vi "FileProducer.vi"(3 "Source File":path=path "C:/ScopeBinaryData.bin", 4 "error in (no error)":errorcluster, 5 "# Channels":i32, 6 "Samples per Channel":i32, 7 "Data Queue":refnum<queue>) -> (0 "error out":errorcluster)   [LabVIEW 2013]
uses:
  Execution Control Global.vi
panel:
  in  "Array":dbl[][](array[numeric])
  out "Data":dbl[][](graph)
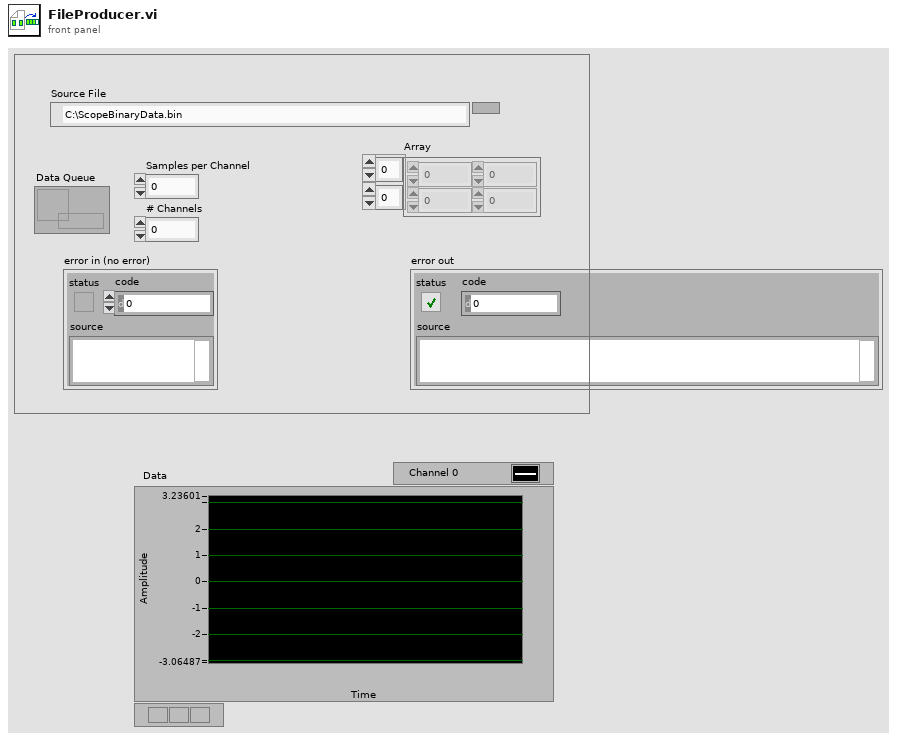
[diagram p1: front panel]
types:
  T1 = enum16{"open", "replace", "create", "open or create", "replace or create", "replace or create with confirmation"}
  T2 = enum16{"big-endian, network order", "native, host order", "little-endian"}
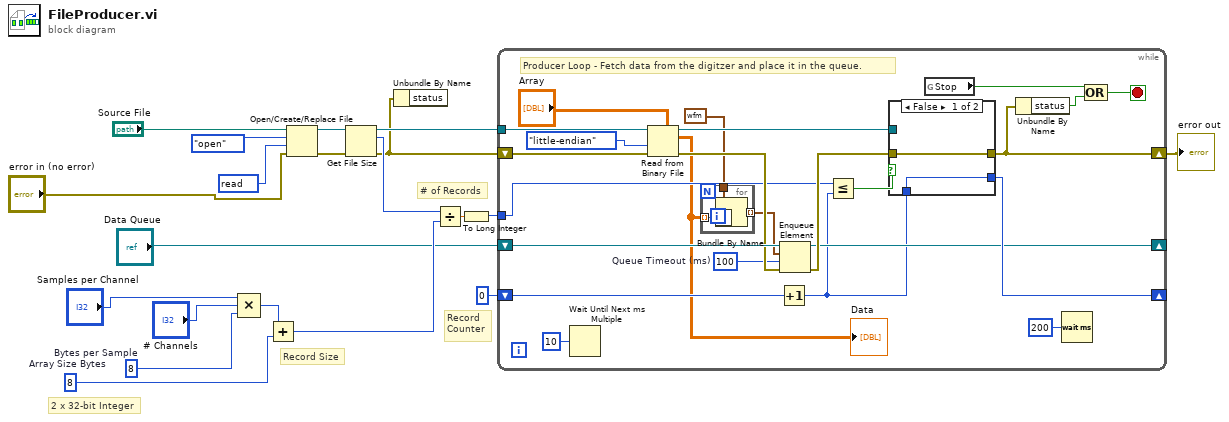
[diagram p0: block diagram]
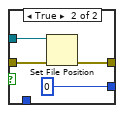
[diagram p2: hidden frame]
diagram:
  w13 = 8  # Array Size Bytes
  w12 = 8  # Bytes per Sample
  w4 = u32 2147483648 items=["read"=2147483648, "write"=1073741824, "read & write"=3221225472, "execute"=536870912, "all"=268435456] ("desired access (read & write)")
  # "# of Records"
  # "Record\nCounter"
  # "Record Size"
  # "2 x 32-bit Integer"
  n1 = Compound Arithmetic op=MULTIPLY("Samples per Channel", "# Channels", w12) -> (w11:i32)
  n2 = Add(x=w11, y=w13) -> (x+y=w10:i32)
  n3 = Open/Create/Replace File(file path (use dialog)="Source File", error in="error in (no error)", operation (0:open)=T1."open", access (0:read/write)=w4) -> (refnum out=w7:refnum<file>, error out=w8:errorcluster)  [unwired: 2 in, 1 out]
  n4 = Get File Size(file=w7, error in=w8) -> (refnum out=w20:refnum<file>, size (in bytes)=w19:i64, 0:w2:errorcluster)
  n5 = Unbundle By Name(w2) -> ()  [unwired: 1 out]
  n6 = Divide(x=w19, y=w10) -> (x/y=w18:dbl)
  n7 = To Long Integer(number=w18) -> (32bit integer=w17:i32)
  n8 = while {
    shift-right: [w40] -> w16
    shift-left: w2 -> [w41]
    tunnel: w20 -> [w42]
    shift-right: [w38] -> _
    shift-left: 0 -> [w26]
    tunnel: w17 -> [w28]
    shift-right: [w34] -> _
    shift-left: "Data Queue" -> [w37]
    stop <- w33 stop-if-true
    w31 = 100  # Queue Timeout (ms)
    # "Producer Loop - Fetch data from the digitzer and place it in the queue."
    n9 = Wait Until Next ms Multiple(millisecond multiple=u32 10) -> ()  [unwired: 1 out]
    n10 = Read from Binary File(5:"Array", 8:w41, 9:T2."little-endian" ("byte order (0:big-endian, network order)"), 11:w42) -> (0:w36:errorcluster, 2:w22:dbl[][], 3:w39:refnum<file>)  [unwired: 2 in, 1 out]
    "Data" <- w22
    n11 = for {
      tunnel: waveform(dbl) {"t0"=timestamp(0 s since 1904-01-01), "dt"=1.0, "Y"=[]} ("Waveform") -> [w47]
      tunnel: w22 -> [w46] mode=indexing
      tunnel: [w45] -> w21 mode=indexing
      n12 = Bundle By Name(cluster=w47, "Y"=w46) -> (w45:waveform(dbl))
    }
    n13 = Increment(x=w26) -> (x+1=w25:i32)
    n14 = Enqueue Element(queue=w37, element=w21, timeout in ms (-1)=w31, error in (no error)=w36) -> (queue out=w34:refnum<queue>, error out=w35:errorcluster)  [unwired: 1 out]
    n15 = Less Or Equal?(x=w28, y=w25) -> (x <= y?=w29:bool)
    n16 = case shown="False" w29 {
      tunnel: w35 -> [w49 w53]
      tunnel: [w49 w52] -> w40
      tunnel: w39 -> [_ w51]
      tunnel: [w48 0] -> w38
      tunnel: w25 -> [w48 _]
      frame False {
      }
      frame True {
        n17 = Set File Position(refnum=w51, error in=w53) -> (error out=w52:errorcluster)  [unwired: 2 in, 1 out]
      }
    }
    n18 = global read "Execution Control Global.vi" "Stop"() -> (w30:bool)
    n19 = Unbundle By Name(w40) -> ("status"=w43:bool)
    n20 = Wait (ms)(milliseconds to wait=u32 200) -> ()  [unwired: 1 out]
    n21 = Compound Arithmetic op=OR(w30, w43) -> (w33:bool)
  }
  "error out" <- w16
